vi "Robot Parameters.vi"() -> ()   [LabVIEW 2011]
panel:
  in  "SubGoal Threshold":dbl=0.5
  in  "Scale (m)":dbl=0.1
  in  "Resolution":i32=200
  in  "LIDAR max range":i32=50000
  in  "max Effort":i32=700
  in  "max RMP":i32=1000
  in  "LIDAR position y":dbl=0.66
  in  "LIDAR position x":dbl
  in  "gear ratio":dbl=1.0
  in  "center of mass y":dbl
  in  "center of mass x":dbl
  in  "robot length":dbl=0.838
  in  "robot width":dbl=0.699
  in  "wheel width":dbl=0.04
  in  "wheel radius":dbl=0.108
  in  "inertia (Izz)":dbl=1.16
  in  "mass":dbl=43.5
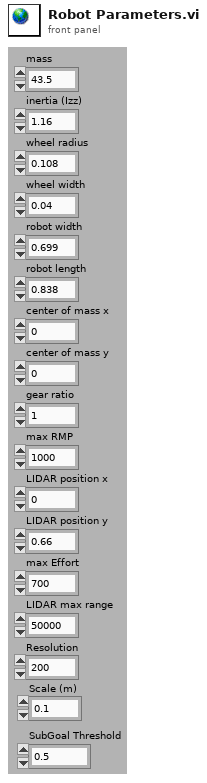
[diagram p1: front panel]
diagram:
